vi "CSM - Drop Broadcast Registry.vi"(11 "Error In":errorcluster caption="error in (no error)") -> (15 "error out":errorcluster)   [LabVIEW 2017, in "Communicable State Machine.lvlib"]
doc: "### CSM - Remove Module in Broadcast Registry.vi\n\n-- <b>Controls</b> --\n- <b>CSM Name</b>:\n\n-- <b>Indicators</b> --\n- <b>CSM Name(dup)</b>:"
uses:
  Communicable State Machine.lvlib
  _Support/FGV-BroadcastRegistry/Operation-BroadcastRegistry.ctl
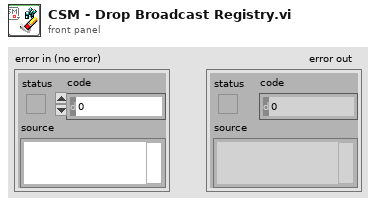
[diagram p1: front panel]
types:
  T1 = typedef "Communicable State Machine.lvlib/Operation-BroadcastRegistry.ctl" = enum16{"Delete Source Module", "Delete Target Module", "Remove Module", "Register", "Unregister", "Check", "List Status", "List Entries", "List Status Of Source", "Drop"}
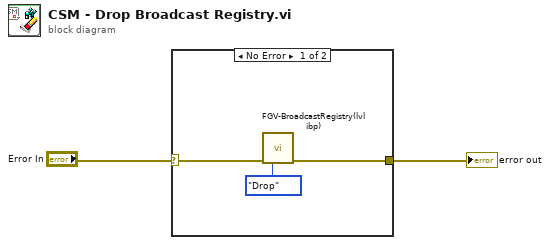
[diagram p0: block diagram]
diagram:
  n1 = case shown="No Error" "Error In" {
    selector: "Error In" -> [w4 w6]
    tunnel: [w3 w6] -> w1
    frame No Error {
      n2 = call "FGV-BroadcastRegistry(lvlibp).vi"("Error In"=w4, "Operation"=Operation-BroadcastRegistry."Drop") -> ("error out"=w3:errorcluster)  [unwired: 12 in, 1 out]
    }
    frame Error {
    }
  }
  "error out" <- w1
